vi "Input Panel.vi"(8 "error in (no error)":errorcluster, 9 "Project in":refnum<class "Project.lvclass">, 11 "Step in":refnum<class "Step.lvclass">) -> (0 "error out":errorcluster, 3 "Step out":refnum<class "Step.lvclass">)   [LabVIEW 2015, in "CallVIStep.lvclass"]
uses:
  CallVIStep.lvclass
  Step.lvclass
  Project.lvclass
  SerializableObject/CONFIGURE_UI_STATE.ctl
  VI Input Control Typedef.ctl
  VI Input Type Typedef.ctl
  Editor/Editor.lvclass
types:
  T1 = typedef "Editor.lvclass/CONFIGURE_UI_STATE.ctl" = enum16{"UI_LOOP", "INIT", "END", "CHANGE_PANEL"}
  T2 = typedef "CallVIStep.lvclass/VI Input Control Typedef.ctl" = cluster{"Ctl Refnum":refnum<vi>, "Input Type":T3, "Value":variant, "Variable Name":string}
  T3 = typedef "CallVIStep.lvclass/VI Input Type Typedef.ctl" = enum16{"Default", "Value", "Variable"}
  T4 = typedef "LVRectTypeDef.ctl" = cluster{"Left":i16, "Top":i16, "Right":i16, "Bottom":i16}
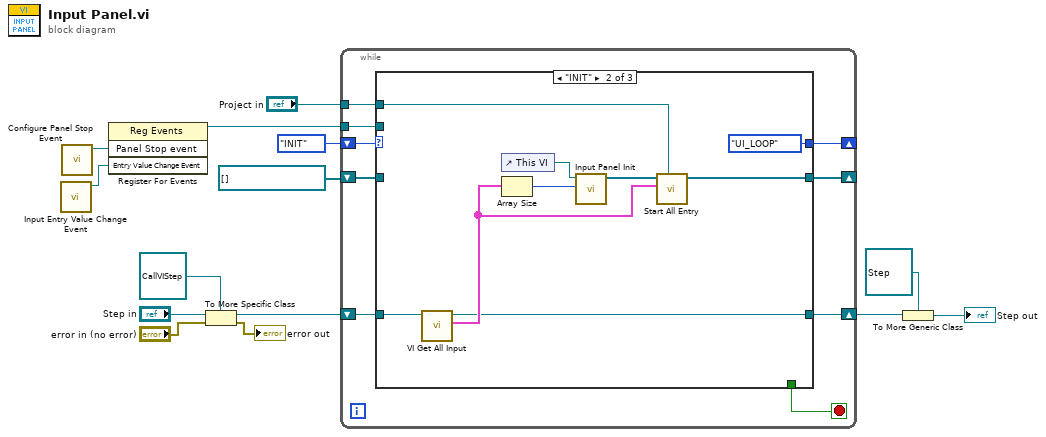
[diagram p0: block diagram]
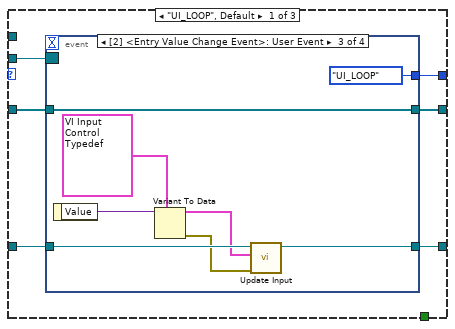
[diagram p2: hidden frame]
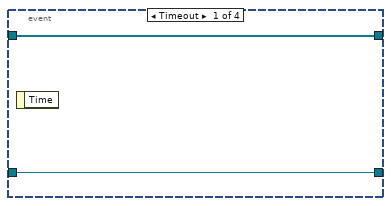
[diagram p3: hidden frame]
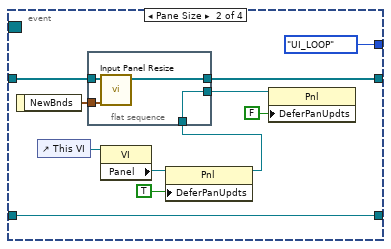
[diagram p4: hidden frame]
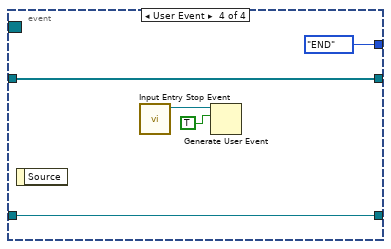
[diagram p5: hidden frame]
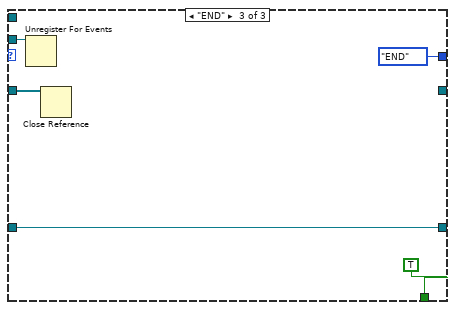
[diagram p6: hidden frame]
diagram:
  n1 = call "Input Entry Value Change Event.vi"() -> ("Entry Value Change Event"=w2:refnum<user-event>)  [unwired: 11 in]
  n2 = call "Configure Panel Stop Event.vi"() -> ("Panel Stop event"=w12:refnum<user-event>)  [unwired: 11 in]
  n3 = register-events(w12, w2) -> (reference out=w11:refnum<event-registration>)  [unwired: 2 in, 1 out]
  n4 = To More Specific Class(target class=refnum<class "CallVIStep.lvclass"> refnum ("CallVIStep in"), reference="Step in", error in="error in (no error)") -> (specific class reference=w4:refnum<class "CallVIStep.lvclass">, error out=→"error out":errorcluster)
  n5 = while {
    shift-right: [w22] -> _
    shift-left: CONFIGURE_UI_STATE."INIT" -> [w23]
    shift-right: [w19] -> _
    shift-left: refnum<vi>[] [] -> [w20]
    tunnel: w11 -> [w18]
    shift-right: [w16] -> w8
    shift-left: w4 -> [w17]
    tunnel: "Project in" -> [w15]
    stop <- w21 stop-if-true
    n6 = case shown="\"INIT\"" w23 {
      tunnel: [w29 CONFIGURE_UI_STATE."UI_LOOP" CONFIGURE_UI_STATE."END"] -> w22
      tunnel: [_ _ TRUE] -> w21
      tunnel: w20 -> [w28 _ w70]
      tunnel: [w27 w64 _] -> w19
      tunnel: w18 -> [w26 _ w71]
      tunnel: w17 -> [w25 w63 w69]
      tunnel: [w24 w61 w69] -> w16
      tunnel: w15 -> [_ w60 _]
      frame "UI_LOOP", Default {
        n7 = event shown="[2] <Entry Value Change Event>: User Event" {
          selector: w26 -> [_ _ _ _]
          dyn-events: _ -> [_ _ _ _]
          timeout: _ -> [_ _ _ _]
          tunnel: [_ CONFIGURE_UI_STATE."UI_LOOP" CONFIGURE_UI_STATE."UI_LOOP" CONFIGURE_UI_STATE."END"] -> w29
          tunnel: w28 -> [w31 w40 w47 w58]
          tunnel: [w31 w39 w47 w58] -> w27
          tunnel: w25 -> [w30 w38 w52 w55]
          tunnel: [w30 w38 w49 w55] -> w24
          event Timeout {
            n8 = event-data() -> ()  [unwired: 1 in, 1 out]
          }
          event Pane Size {
            n9 = event-data() -> ("NewBnds"=w41:T4)  [unwired: 1 in]
            n10 = control-ref of="This VI"() -> (w37:refnum<vi>)
            n11 = flat-sequence {
              tunnel: w41 -> [w46]
              tunnel: w40 -> [w45]
              tunnel: [w44] -> w39
              tunnel: w34 -> [w43]
              tunnel: [w43] -> w33
              frame #0 {
                n12 = call "Input Panel Resize.vi"("NewBnds"=w46, "Entry Panel in"=w45) -> ("Entry Panel out"=w44:refnum<vi>[])  [unwired: 9 in]
              }
            }
            n13 = property class="VI"(reference=w37) -> ("Panel"=w36:refnum<vi>)  [unwired: 1 in, 2 out]
            n14 = property class="Pnl"(reference=w36, "DeferPanUpdts"=TRUE ("Defer Panel Updates")) -> (reference out=w34:refnum<vi>)  [unwired: 1 in, 1 out]
            n15 = property class="Pnl"(reference=w33, "DeferPanUpdts"=FALSE ("Defer Panel Updates")) -> ()  [unwired: 1 in, 2 out]
          }
          event User Event {
            n16 = event-data() -> ("Value"=w54:variant)  [unwired: 1 in]
            n17 = Variant To Data(type=T2 {"Ctl Refnum"=refnum, "Input Type"=enum."Default", "Value"=variant, "Variable Name"=""} ("Input Control"), Variant=w54) -> (data=w51:T2, error out=w50:errorcluster)  [unwired: 1 in]
            n18 = call-dynamic "Update Input.vi"("error in (no error)"=w50, "Input Control"=w51, "CallVIStep in"=w52) -> ("CallVIStep out"=w49:refnum<class "CallVIStep.lvclass">)  [unwired: 7 in, 1 out]
          }
          event User Event {
            n19 = event-data() -> ()  [unwired: 1 in, 1 out]
            n20 = call "Input Entry Stop Event.vi"() -> ("Entry Stop event"=w57:refnum<user-event>)  [unwired: 11 in]
            n21 = Generate User Event(user event=w57, event data cluster=TRUE ("event data")) -> ()  [unwired: 2 in, 2 out]
          }
        }
      }
      frame "INIT" {
        n22 = call-dynamic "VI Get All Input.vi"("CallVIStep in"=w63) -> ("Input Control"=w62:T2[], "CallVIStep out"=w61:refnum<class "CallVIStep.lvclass">)  [unwired: 8 in, 1 out]
        n23 = control-ref of="This VI"() -> (w67:refnum<vi>)
        n24 = Array Size(array=w62) -> (size(s)=w66:i32)
        n25 = call "Input Panel Init.vi"("Size"=w66, "VI in"=w67) -> ("Entry Panel out"=w65:refnum<vi>[])  [unwired: 8 in, 1 out]
        n26 = call "Start All Entry.vi"("Project In"=w60, "Input Control"=w62, "Entry Panel in"=w65) -> ("Entry Panel out"=w64:refnum<vi>[])  [unwired: 6 in, 2 out]
      }
      frame "END" {
        n27 = Unregister For Events(event registration refnum=w71) -> ()  [unwired: 1 in, 1 out]
        n28 = Close Reference(reference=w70) -> ()  [unwired: 1 in, 1 out]
      }
    }
  }
  n29 = To More Generic Class(target class=refnum<class "Step.lvclass"> refnum ("CallVIStep in"), reference=w8) -> (generic class reference=→"Step out":refnum<class "Step.lvclass">)
